vi "Example.vi"() -> ()   [LabVIEW 2012]
uses:
  Conditional Increment VIs/Conditional Increment - I32.vi
  femtoRoboLib.lvlib
panel:
  in  "Round To":dbl=12.0
  out "Output":dbl
  in  "Input":dbl=27.0
  out "Conditional Incrementing":i32
  out "Trailing":bool
  out "Leading":bool
  out "Start Trigger":bool
  out "End Trigger":bool
  out "Timer Running":bool
  out "Button Out":bool
  in  "Delay":u32=1000
  in  "Mode":enum16{"Noop", "Button", "Switch"}(ring)=enum."Switch"
  in  "Button":bool
  in  "Reset":bool
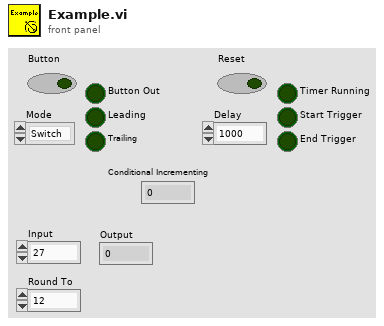
[diagram p1: front panel]
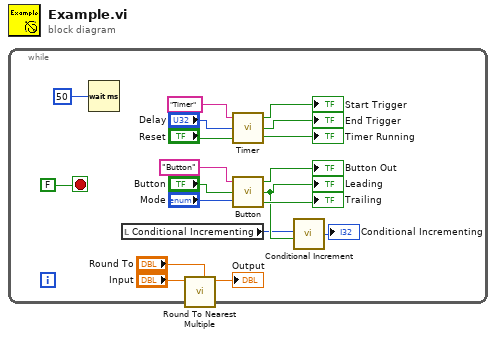
[diagram p0: block diagram]
diagram:
  n1 = while {
    stop <- FALSE stop-if-true
    n2 = Wait (ms)(milliseconds to wait=u32 50) -> ()  [unwired: 1 out]
    n3 = local read "Conditional Incrementing"() -> (w4:i32)
    n4 = call "Round To Nearest Multiple.vi"("Round To"="Round To", "Input"="Input") -> ("Output"=→"Output":dbl)  [unwired: 9 in]
    n5 = call "Timer.vi"("Reset"="Reset", "Delay"="Delay", "Name"="Timer") -> ("Running"=→"Timer Running":bool, "End Trigger"=→"End Trigger":bool, "Start Trigger"=→"Start Trigger":bool)
    n6 = call "Button.vi"("Set Mode"="Mode", "In"="Button", "Name"="Button") -> ("Trailing"=→"Trailing":bool, "Leading"=w6:bool, "Out"=→"Button Out":bool)
    "Leading" <- w6
    n7 = call-poly "Conditional Increment.vi"("Condition"=w6, "Input"=w4) -> ("Output"=→"Conditional Incrementing":i32)  [unwired: 2 in]
  }
